vi "运动学逆解.vi"(2 "逆运动学输入":dbl[](array[numeric])=[993.0, 0.0, 902.0], 3 "机械臂末端姿态":dbl[][](array[numeric])=[[1.0, 0.0, 0.0], [0.0, 1.0, 0.0], [0.0, 0.0, 1.0]]) -> (0 "运动学逆解2":dbl[](array[numeric]), 1 "运动学逆解1":dbl[](array[numeric]))   [LabVIEW 2015]
panel:
  out "ans4":dbl[](array[numeric])=[0.0, 90.0, 0.0, 0.0, -90.0, -0.0] format="%#.3f"
  out "ans3":dbl[](array[numeric])=[0.0, 90.0, 0.0, 0.0, -90.0, -0.0] format="%#.3f"
  out "ans2":dbl[](array[numeric])=[0.0, 90.0, 0.0, 0.0, -90.0, -0.0] format="%#.3f"
  out "ans1":dbl[](array[numeric])=[0.0, 90.0, 0.0, 0.0, -90.0, -0.0] format="%#.3f"
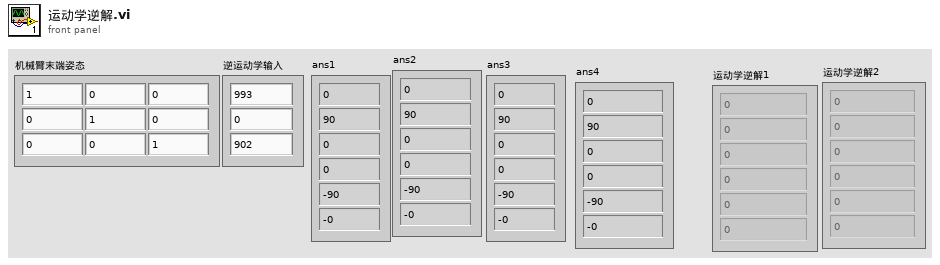
[diagram p1: front panel]
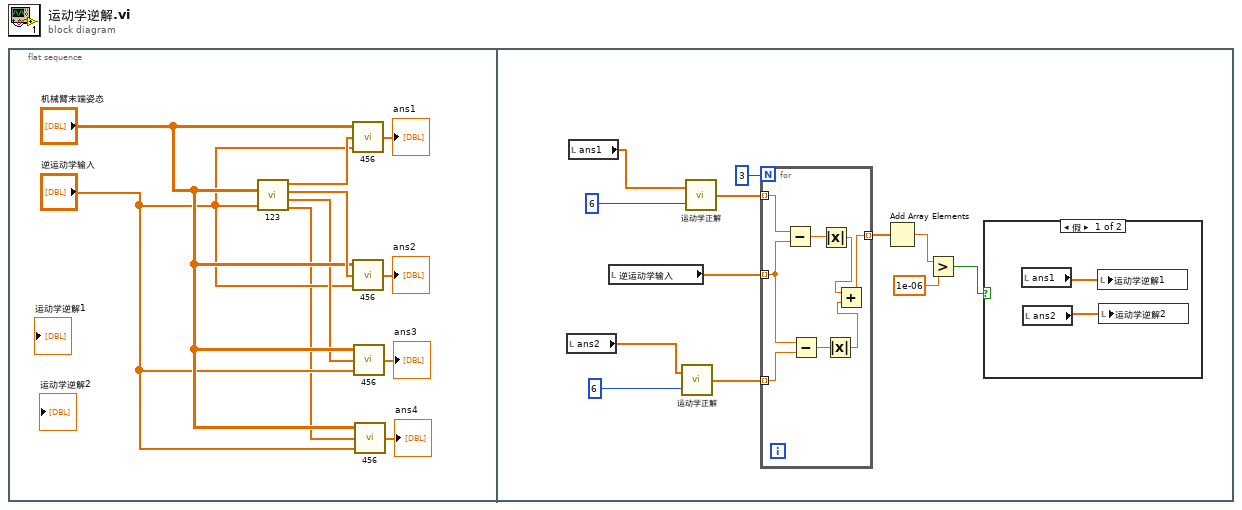
[diagram p0: block diagram]
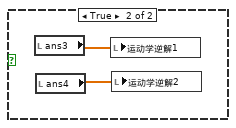
[diagram p2: hidden frame]
diagram:
  n1 = flat-sequence {
    frame #0 {
      n2 = call "123.vi"("机械臂末端姿态"="机械臂末端姿态", "逆运动学输入"="逆运动学输入") -> ("1231"=w10:dbl[], "1232"=w8:dbl[], "1233"=w5:dbl[], "1234"=w3:dbl[])
      n3 = call "456.vi"("逆运动学输入"="逆运动学输入", "123"=w10, "机械臂末端姿态"="机械臂末端姿态") -> ("逆运动学输出"=→"ans1":dbl[])
      n4 = call "456.vi"("逆运动学输入"="逆运动学输入", "123"=w8, "机械臂末端姿态"="机械臂末端姿态") -> ("逆运动学输出"=→"ans2":dbl[])
      n5 = call "456.vi"("逆运动学输入"="逆运动学输入", "123"=w5, "机械臂末端姿态"="机械臂末端姿态") -> ("逆运动学输出"=→"ans3":dbl[])
      n6 = call "456.vi"("逆运动学输入"="逆运动学输入", "123"=w3, "机械臂末端姿态"="机械臂末端姿态") -> ("逆运动学输出"=→"ans4":dbl[])
    }
    frame #1 {
      n7 = local read "ans2"() -> (w13:dbl[])
      n8 = local read "ans1"() -> (w22:dbl[])
      n9 = local read "逆运动学输入"() -> (w18:dbl[])
      n10 = call "运动学正解.vi"("正运动学输入"=w13, "关节数"=6) -> ("正解输出"=w11:dbl[])  [unwired: 2 out]
      n11 = call "运动学正解.vi"("正运动学输入"=w22, "关节数"=6) -> ("正解输出"=w19:dbl[])  [unwired: 2 out]
      n12 = for {
        N: 3 -> [_]
        tunnel: w19 -> [w34] mode=indexing
        tunnel: w18 -> [w32] mode=indexing
        tunnel: [w27] -> w17 mode=indexing
        tunnel: w11 -> [w31] mode=indexing
        n13 = Subtract(x=w34, y=w32) -> (x-y=w33:dbl)
        n14 = Subtract(x=w32, y=w31) -> (x-y=w30:dbl)
        n15 = Absolute Value(x=w33) -> (abs(x)=w28:dbl)
        n16 = Absolute Value(x=w30) -> (abs(x)=w29:dbl)
        n17 = Add(x=w28, y=w29) -> (x+y=w27:dbl)
      }
      n18 = Add Array Elements(numeric array=w17) -> (sum=w16:dbl)
      n19 = Greater?(x=w16, y=1e-06) -> (0:w14:bool)
      n20 = case shown="假" w14 {
        frame False {
          n21 = local read "ans1"() -> (w24:dbl[])
          n22 = local read "ans2"() -> (w23:dbl[])
          n23 = local write "运动学逆解1"(w24) -> ()
          n24 = local write "运动学逆解2"(w23) -> ()
        }
        frame True {
          n25 = local read "ans3"() -> (w26:dbl[])
          n26 = local read "ans4"() -> (w25:dbl[])
          n27 = local write "运动学逆解1"(w26) -> ()
          n28 = local write "运动学逆解2"(w25) -> ()
        }
      }
    }
  }
